vi "Get all Object Items.vi"(8 "error in (no error)":errorcluster, 10 "Offset":i32, 11 "JSON":string) -> (0 "error out":errorcluster, 1 "<JSON>":string[](array[string]) caption="<JSON>Items", 2 "Offset past":i32 caption="Offset past Object", 3 "Item Names":string[](array[string]))   [LabVIEW 2021, in "json.facade.lvlib"]
doc: "Return all Items in the Object as an array of JSON Values."
uses:
  json.facade.lvlib
  jsontext/JSONtext.lvlib
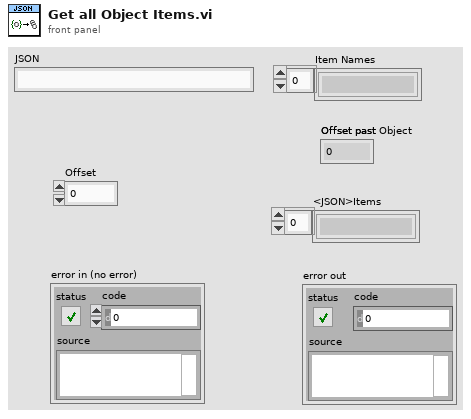
[diagram p1: front panel]
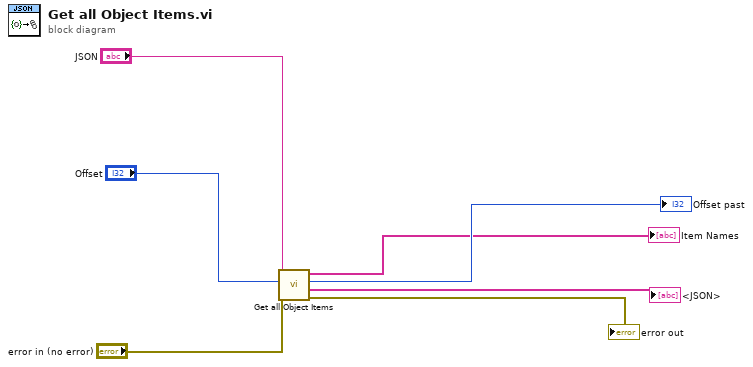
[diagram p0: block diagram]
diagram:
  n1 = call "Get all Object Items.vi"("error in (no error)"="error in (no error)", "Offset"="Offset", "JSON"="JSON") -> ("error out"=→"error out":errorcluster, "<JSON>"=→"<JSON>":string[], "Offset past"=→"Offset past":i32, "Item Names"=→"Item Names":string[])  [unwired: 5 in]
